vi "Shooter LED Control.vi"(0 "Current Shooter Speed":dbl, 1 "Shooter Shooting":bool, 2 "Shooter SP":dbl) -> (7 "Shooter LED Send":string)   [LabVIEW 2016]
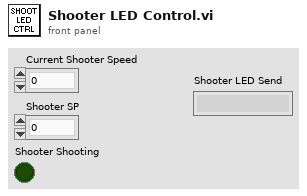
[diagram p1: front panel]
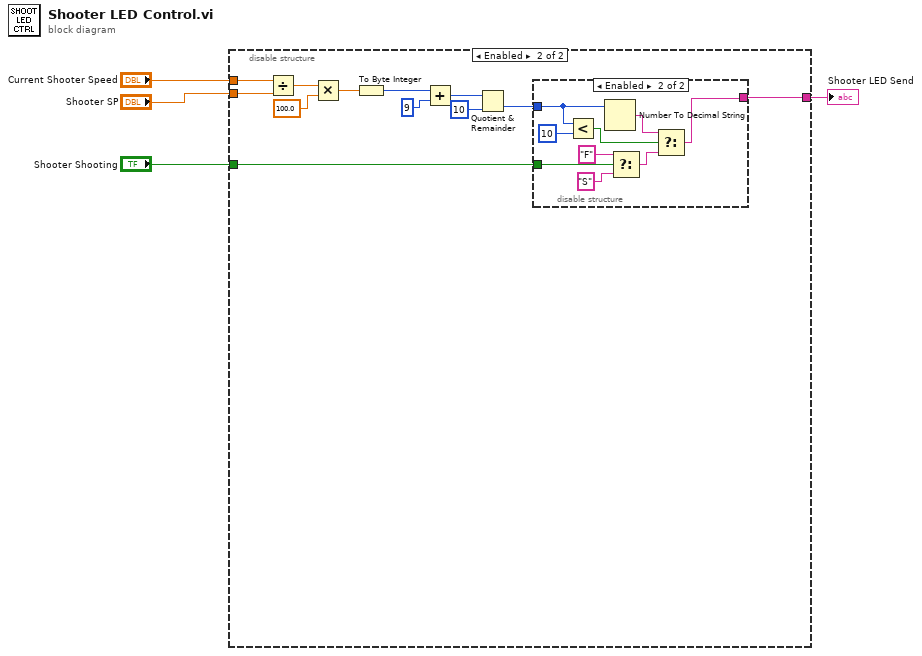
[diagram p0: block diagram]
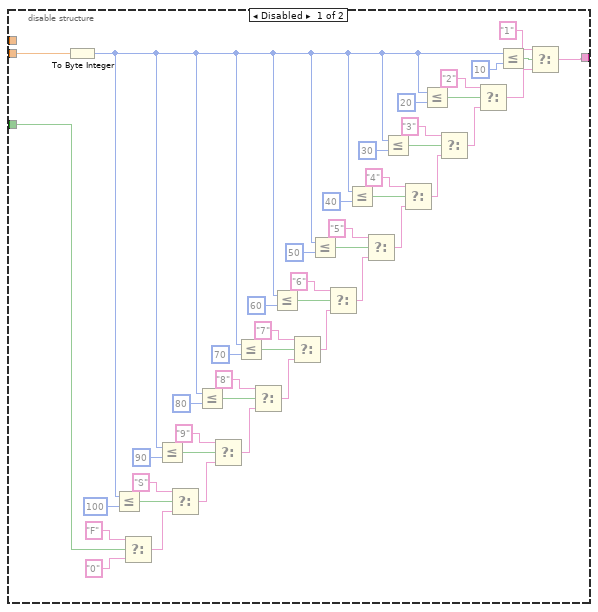
[diagram p2: hidden frame]
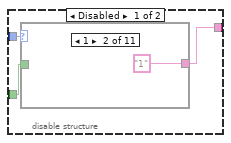
[diagram p3: hidden frame]
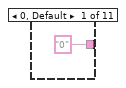
[diagram p4: hidden frame]
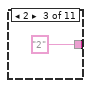
[diagram p5: hidden frame]
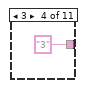
[diagram p6: hidden frame]
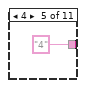
[diagram p7: hidden frame]
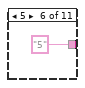
[diagram p8: hidden frame]
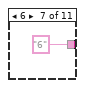
[diagram p9: hidden frame]
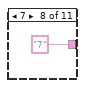
[diagram p10: hidden frame]
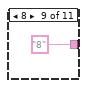
[diagram p11: hidden frame]
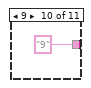
[diagram p12: hidden frame]
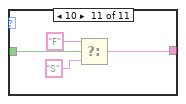
[diagram p13: hidden frame]
diagram:
  n1 = disable-structure shown="Enabled" {
    disable-tunnel: [w43 w52] -> w4
    disable-tunnel: "Shooter SP" -> [w8 w59]
    disable-tunnel: "Shooter Shooting" -> [w6 w51]
    disable-tunnel: "Current Shooter Speed" -> [_ w58]
    frame Disabled {
      n2 = To Byte Integer(number=w8) -> (8bit integer=w5:i8)
      n3 = Less Or Equal?(x=w5, y=i8 100) -> (x <= y?=w13:bool)
      n4 = Select(t="F", s=w6, f="0") -> (s? t:f=w10:string)
      n5 = Less Or Equal?(x=w5, y=i8 90) -> (x <= y?=w17:bool)
      n6 = Select(t="S", s=w13, f=w10) -> (s? t:f=w12:string)
      n7 = Less Or Equal?(x=w5, y=i8 80) -> (x <= y?=w21:bool)
      n8 = Select(t="9", s=w17, f=w12) -> (s? t:f=w16:string)
      n9 = Less Or Equal?(x=w5, y=i8 70) -> (x <= y?=w25:bool)
      n10 = Select(t="8", s=w21, f=w16) -> (s? t:f=w19:string)
      n11 = Less Or Equal?(x=w5, y=i8 60) -> (x <= y?=w29:bool)
      n12 = Select(t="7", s=w25, f=w19) -> (s? t:f=w24:string)
      n13 = Less Or Equal?(x=w5, y=i8 50) -> (x <= y?=w33:bool)
      n14 = Select(t="6", s=w29, f=w24) -> (s? t:f=w28:string)
      n15 = Less Or Equal?(x=w5, y=i8 40) -> (x <= y?=w37:bool)
      n16 = Select(t="5", s=w33, f=w28) -> (s? t:f=w32:string)
      n17 = Less Or Equal?(x=w5, y=i8 30) -> (x <= y?=w41:bool)
      n18 = Select(t="4", s=w37, f=w32) -> (s? t:f=w36:string)
      n19 = Less Or Equal?(x=w5, y=i8 20) -> (x <= y?=w46:bool)
      n20 = Select(t="3", s=w41, f=w36) -> (s? t:f=w40:string)
      n21 = Select(t="2", s=w46, f=w40) -> (s? t:f=w45:string)
      n22 = Less Or Equal?(x=w5, y=i8 10) -> (x <= y?=w50:bool)
      n23 = Select(t="1", s=w50, f=w45) -> (s? t:f=w43:string)
    }
    frame Enabled {
      n24 = Divide(x=w58, y=w59) -> (x/y=w62:dbl)
      n25 = Multiply(x=w62, y=100.0) -> (x*y=w60:dbl)
      n26 = To Byte Integer(number=w60) -> (8bit integer=w57:i8)
      n27 = Add(x=w57, y=i8 9) -> (x+y=w54:i8)
      n28 = Quotient & Remainder(x=w54, y=i8 10) -> (floor(x/y)=w55:i8)  [unwired: 1 out]
      n29 = disable-structure shown="Enabled" {
        disable-tunnel: w55 -> [w65 w87]
        disable-tunnel: [w64 w81] -> w52
        disable-tunnel: w51 -> [w63 w83]
        frame Disabled {
          n30 = case shown="1" w65 {
            tunnel: ["0" "1" "2" "3" "4" "5" "6" "7" "8" "9" w78] -> w64
            tunnel: w63 -> [_ _ _ _ _ _ _ _ _ _ w79]
            frame 0, Default {
            }
            frame 1 {
            }
            frame 2 {
            }
            frame 3 {
            }
            frame 4 {
            }
            frame 5 {
            }
            frame 6 {
            }
            frame 7 {
            }
            frame 8 {
            }
            frame 9 {
            }
            frame 10 {
              n31 = Select(t="F", s=w79, f="S") -> (s? t:f=w78:string)
            }
          }
        }
        frame Enabled {
          n32 = Less?(x=w87, y=i8 10) -> (x < y?=w85:bool)
          n33 = Number To Decimal String(number=w87) -> (decimal integer string=w86:string)  [unwired: 1 in]
          n34 = Select(t="F", s=w83, f="S") -> (s? t:f=w82:string)
          n35 = Select(t=w86, s=w85, f=w82) -> (s? t:f=w81:string)
        }
      }
    }
  }
  "Shooter LED Send" <- w4
